vi "ParaStack.vi"(0 "StartPos":dbl[](array[numeric]), 1 "Direction":enum16{"Y to X", "X to Y"}(ring), 2 "LineNo":i32, 4 "MinJT":dbl, 5 "Vel":dbl, 6 "MaxJT":dbl, 7 "Length":dbl, 9 "Acc":dbl, 11 "error in":errorcluster, 12 "StackNo":i32, 13 "Spacing":dbl) -> (15 "error out":errorcluster)   [LabVIEW 2022 SP3]
uses:
  Newport.XPS.CommandInterface
  Global 3.vi
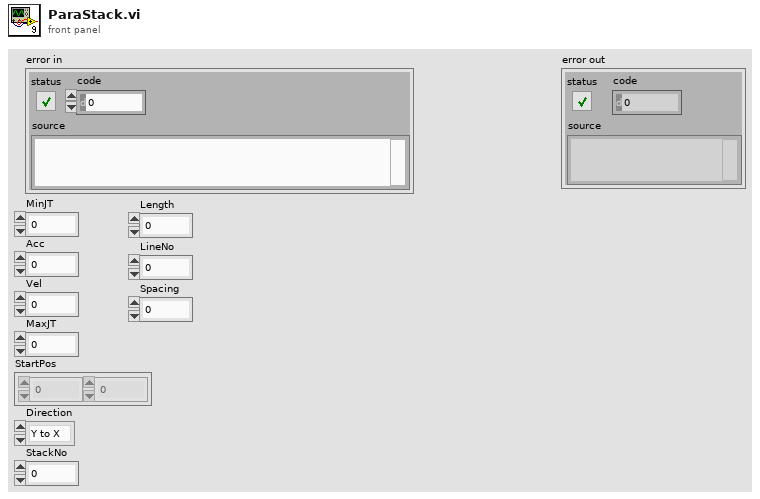
[diagram p1: front panel]
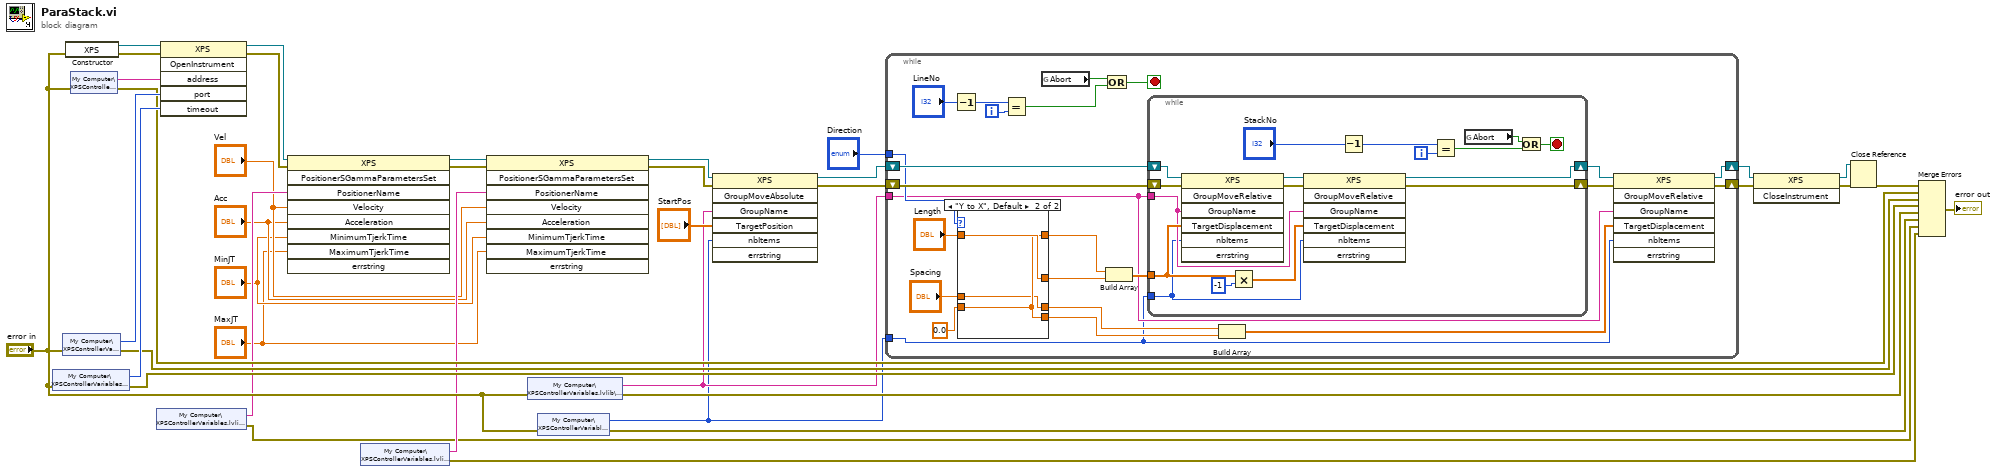
[diagram p0: block diagram]
diagram:
  n1 = shared-variable "My Computer\\XPSControllerVariables.lvlib\\Timeout"(error in="error in") -> (w33:i16, error out=w28:errorcluster)
  n2 = shared-variable "My Computer\\XPSControllerVariables.lvlib\\Port"(error in="error in") -> (w34:i16, error out=w29:errorcluster)
  n3 = constructor class="XPS"(error in="error in") -> (reference out=w37:refnum<k24>, error out=w36:errorcluster)  [unwired: 2 in, 1 out]
  n4 = shared-variable "My Computer\\XPSControllerVariables.lvlib\\IP"(error in="error in") -> (w35:string, error out=w30:errorcluster)
  n5 = shared-variable "My Computer\\XPSControllerVariables.lvlib\\PosNameX"() -> (w16:string, error out=w9:errorcluster)  [unwired: 1 in]
  n6 = invoke class="XPS" method="OpenInstrument"(reference=w37, error in=w36, "address"=w35, "port"=w34, "timeout"=w33) -> (reference out=w22:refnum<k24>, error out=w21:errorcluster)  [unwired: 1 in, 4 out]
  n7 = invoke class="XPS" method="PositionerSGammaParametersSet"(reference=w22, error in=w21, "PositionerName"=w16, "Velocity"="Vel", "Acceleration"="Acc", "MinimumTjerkTime"="MinJT", "MaximumTjerkTime"="MaxJT") -> (reference out=w20:refnum<k24>, error out=w19:errorcluster)  [unwired: 2 in, 7 out]
  n8 = shared-variable "My Computer\\XPSControllerVariables.lvlib\\PosNameY"() -> (w15:string, error out=w8:errorcluster)  [unwired: 1 in]
  n9 = invoke class="XPS" method="PositionerSGammaParametersSet"(reference=w20, error in=w19, "PositionerName"=w15, "Velocity"="Vel", "Acceleration"="Acc", "MinimumTjerkTime"="MinJT", "MaximumTjerkTime"="MaxJT") -> (reference out=w18:refnum<k24>, error out=w17:errorcluster)  [unwired: 2 in, 7 out]
  n10 = shared-variable "My Computer\\XPSControllerVariables.lvlib\\GroupName"(error in="error in") -> (w3:string, error out=w27:errorcluster)
  n11 = shared-variable "My Computer\\XPSControllerVariables.lvlib\\nbitem"(error in="error in") -> (w2:i16, error out=w23:errorcluster)
  n12 = invoke class="XPS" method="GroupMoveAbsolute"(reference=w18, error in=w17, "GroupName"=w3, "TargetPosition"="StartPos", "nbItems"=w2) -> (reference out=w7:refnum<k24>, error out=w6:errorcluster)  [unwired: 2 in, 5 out]
  n13 = while {
    tunnel: w3 -> [w39]
    tunnel: w2 -> [w38]
    shift-right: [w43] -> w5
    shift-left: w7 -> [w61]
    shift-right: [w42] -> w4
    shift-left: w6 -> [w60]
    tunnel: "Direction" -> [w46]
    i -> [w57]
    stop <- w54 stop-if-true
    n14 = Decrement(x="LineNo") -> (x-1=w58:i32)
    n15 = case shown="\"Y to X\", Default" w46 {
      tunnel: [w81 w83] -> w53
      tunnel: "Length" -> [w81 w84]
      tunnel: [w80 w84] -> w51
      tunnel: 0.0 -> [w80 w83]
      tunnel: [w80 w82] -> w49
      tunnel: [w79 w83] -> w48
      tunnel: "Spacing" -> [w79 w82]
      frame "X to Y" {
      }
      frame "Y to X", Default {
      }
    }
    n16 = Equal?(x=w58, y=w57) -> (x = y?=w55:bool)
    n17 = global read "Global 3.vi" "Abort"() -> (w56:bool)
    n18 = Or(x=w56, y=w55) -> (x .or. y?=w54:bool)
    n19 = Build Array(w53, w51) -> (w40:dbl[])
    n20 = while {
      tunnel: w40 -> [w72]
      tunnel: w39 -> [w69]
      tunnel: w38 -> [w68]
      shift-right: [w74] -> w45
      shift-left: w61 -> [w78]
      shift-right: [w73] -> w44
      shift-left: w60 -> [w77]
      i -> [w65]
      stop <- w62 stop-if-true
      n21 = invoke class="XPS" method="GroupMoveRelative"(reference=w78, error in=w77, "GroupName"=w69, "TargetDisplacement"=w72, "nbItems"=w68) -> (reference out=w76:refnum<k24>, error out=w75:errorcluster)  [unwired: 2 in, 5 out]
      n22 = Multiply(x=w72, y=-1) -> (x*y=w70:dbl[])
      n23 = invoke class="XPS" method="GroupMoveRelative"(reference=w76, error in=w75, "GroupName"=w69, "TargetDisplacement"=w70, "nbItems"=w68) -> (reference out=w74:refnum<k24>, error out=w73:errorcluster)  [unwired: 2 in, 5 out]
      n24 = Decrement(x="StackNo") -> (x-1=w66:i32)
      n25 = Equal?(x=w66, y=w65) -> (x = y?=w64:bool)
      n26 = global read "Global 3.vi" "Abort"() -> (w63:bool)
      n27 = Or(x=w63, y=w64) -> (x .or. y?=w62:bool)
    }
    n28 = Build Array(w49, w48) -> (w41:dbl[])
    n29 = invoke class="XPS" method="GroupMoveRelative"(reference=w45, error in=w44, "GroupName"=w39, "TargetDisplacement"=w41, "nbItems"=w38) -> (reference out=w43:refnum<k24>, error out=w42:errorcluster)  [unwired: 2 in, 5 out]
  }
  n30 = invoke class="XPS" method="CloseInstrument"(reference=w5, error in=w4) -> (reference out=w32:refnum<k24>, error out=w31:errorcluster)  [unwired: 1 in, 1 out]
  n31 = Close Reference(reference=w32, error in (no error)=w31) -> (error out=w26:errorcluster)
  n32 = Merge Errors(w26, w30, w29, w28, w27, w23, w9, w8) -> (→"error out":errorcluster)
